vi "Pipe Var Intf - Read Data ACK.vi"(7 "timeout [ms]":i32=3000, 8 "error in (no error)":errorcluster, 10 "read count":u32, 11 "pipe handle":i32) -> (0 "error out":errorcluster, 1 "data count":i32, 2 "data out":u8[](array[numeric]), 3 "pipe handle out":i32)   [LabVIEW 2020, in "GOLPI library.lvlib"]
doc: "Tries to read data via Pipe Variable Interface with ACK to sender after every transfered data block. Note this is workaround for pipe fail when trying to transfer lot of data. I was not able to identify why the pipe closes. It does not do that in the other direction."
uses:
  GOLPI library.lvlib
  <vilib>/Utility/error.llb/Error Cluster From Error Code.vi
  <vilib>/ErrorRing/Error Ring.xnode
panel:
  out "timeout remain [ms]":dbl
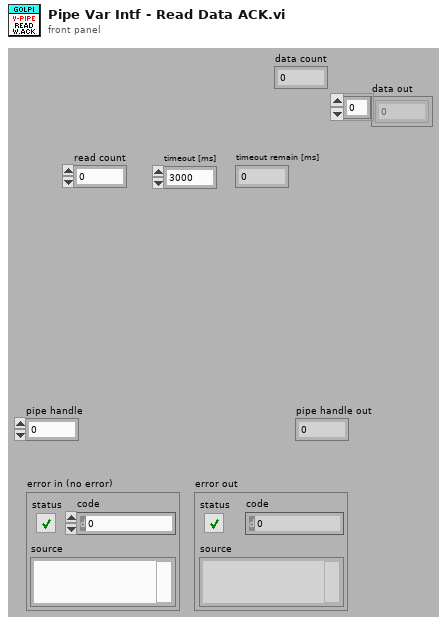
[diagram p1: front panel]
types:
  T1 = enum16{"big-endian, network order", "native, host order", "little-endian"}
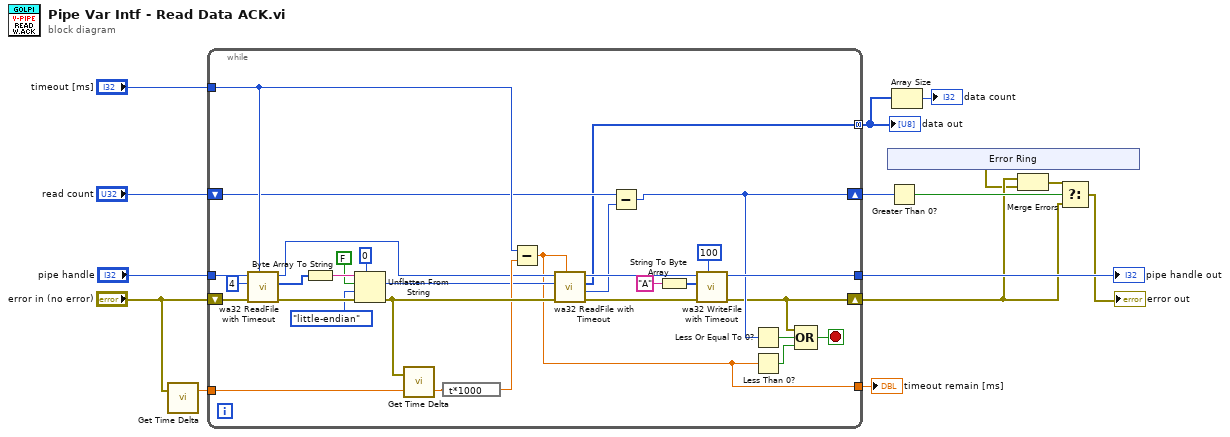
[diagram p0: block diagram]
diagram:
  n1 = call "Get Time Delta.vi"("anything in (for synchronization)"="error in (no error)") -> ("time now"=w12:dbl)  [unwired: 1 in, 1 out]
  n2 = while {
    tunnel: [w38] -> w15
    tunnel: "pipe handle" -> [w37]
    tunnel: w12 -> [w35]
    tunnel: "timeout [ms]" -> [w33]
    shift-right: [w21] -> w6
    shift-left: "error in (no error)" -> [w36]
    shift-right: [w22] -> w9
    shift-left: "read count" -> [w23]
    tunnel: [w17] -> w3 mode=concatenating
    tunnel: [w16] -> w1
    stop <- w18 stop-if-true
    n3 = call "wa32 ReadFile with Timeout.vi"("timeout [ms]"=w33, "error in (no error)"=w36, "read count (0: all)"=4, "pipe handle"=w37) -> ("error out"=w45:errorcluster, "data out"=w44:u8[], "pipe handle out"=w30:i32)  [unwired: 4 in, 1 out]
    n4 = Byte Array To String(unsigned byte array=w44) -> (string=w43:string)
    n5 = Unflatten From String(type=0, binary string=w43, data includes array or string size? (T)=FALSE, byte order (0:big-endian, network order)=T1."little-endian", error in (no error)=w45) -> (value=w29:i32, error out=w34:errorcluster)  [unwired: 1 out]
    n6 = call "Get Time Delta.vi"("reference time (0)"=w35, "anything in (for synchronization)"=w34) -> ("time delta [s]"=w32:dbl)  [unwired: 1 out]
    n7 = expression code="t*1000"(w32) -> (w31:dbl)
    n8 = Subtract(x=w33, y=w31) -> (x-y=w16:dbl)
    n9 = call "wa32 ReadFile with Timeout.vi"("timeout [ms]"=w16, "error in (no error)"=w34, "read count (0: all)"=w29, "pipe handle"=w30) -> ("error out"=w28:errorcluster, "read count"=w24:u32, "data out"=w17:u8[], "pipe handle out"=w27:i32)  [unwired: 4 in]
    n10 = Subtract(x=w23, y=w24) -> (x-y=w22:u32)
    n11 = String To Byte Array(string="A") -> (unsigned byte array=w25:u8[])
    n12 = call "wa32 WriteFile with Timeout.vi"("timeout [ms]"=100, "error in (no error)"=w28, "data"=w25, "pipe handle"=w27) -> ("error out"=w21:errorcluster, "pipe handle out"=w38:i32)  [unwired: 5 in, 1 out]
    n13 = Less Or Equal To 0?(x=w22) -> (x <= 0?=w20:bool)
    n14 = Less Than 0?(x=w16) -> (x < 0?=w19:bool)
    n15 = Compound Arithmetic op=OR(w21, w20, w19) -> (w18:bool)
  }
  "pipe handle out" <- w15
  "data out" <- w3
  "timeout remain [ms]" <- w1
  n16 = xnode "Error Ring"() -> ("error out"=w5:errorcluster)
  n17 = Greater Than 0?(x=w9) -> (x > 0?=w8:bool)
  n18 = Array Size(array=w3) -> (size(s)=→"data count":i32)
  n19 = Merge Errors(w6, w5) -> (w7:errorcluster)
  n20 = Select(t=w7, s=w8, f=w6) -> (s? t:f=→"error out":errorcluster)
